vi "Events.vi"(8 "error in (no error)":errorcluster, 11 "EventHandler in":refnum<class "EventHandler.lvclass">) -> (0 "error out":errorcluster, 2 "Events":T1[](array[typedef]), 3 "EventHandler out":refnum<class "EventHandler.lvclass">)   [LabVIEW 2020, in "Volatus.lvlib" / "EventHandler.lvclass"]
uses:
  EventHandler.lvclass
  Event.ctl
  Event Level.ctl
  Volatus.lvlib
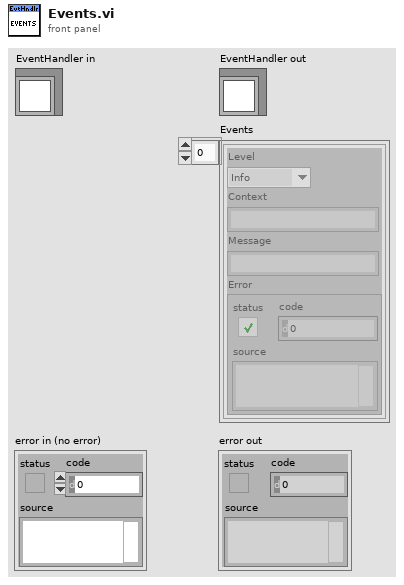
[diagram p1: front panel]
types:
  T1 = typedef "Volatus.lvlib/Event.ctl" = cluster{"Level":T2, "Context":string, "Message":string, "Error":errorcluster}
  T2 = typedef "Volatus.lvlib/Event Level.ctl" = enum16{"Debug", "Info", "Warning", "Error"}
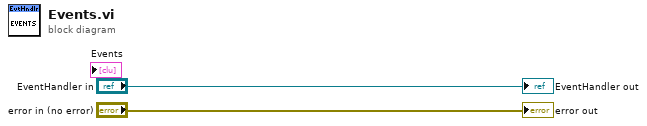
[diagram p0: block diagram]
diagram:
  "error out" <- "error in (no error)"
  "EventHandler out" <- "EventHandler in"
